vi "Save ALL Contacts.vi"(6 "Command":T8=enum."Set Position", 8 "error in (no error)":errorcluster, 11 "Contact in":T1[](array[typedef])) -> (0 "error out":errorcluster, 3 "Contact out":T1[](array[typedef]))   [LabVIEW 2014, in "Contact Data.lvlib"]
doc: "Updates an existing contact or inserts a new contact into the address book data store. Use the ID of an existing contact to update, or an ID of 0 to insert. When inserting, the output cluster will contain the ID of the new contact."
uses:
  Contact Data.lvlib
  Command.ctl
  Contact.ctl
  Position.ctl
  Controls.ctl
  DestinationCluster.ctl
  DesinationControls.ctl
  PathData.ctl
  Components/PathFinder/Controls/PathControl.ctl
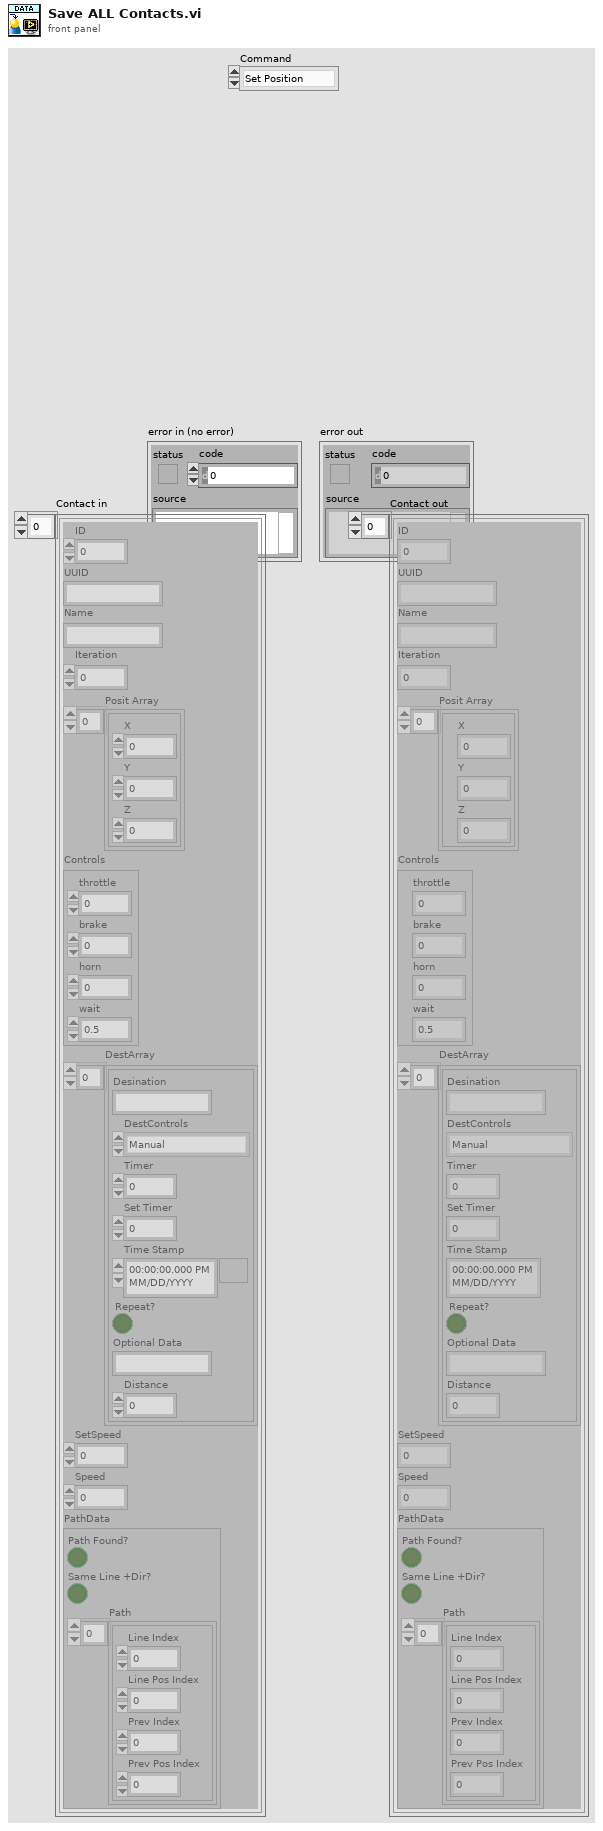
[diagram p1: front panel]
types:
  T1 = typedef "Contact Data.lvlib/Contact.ctl" = cluster{"ID":u32, "UUID":string, "Name":string, "Iteration":i32, "Posit Array":T2[], "Controls":T3, "DestArray":T4[], "SetSpeed":dbl, "Speed":dbl, "PathData":T6}
  T2 = typedef "Contact Data.lvlib/Position.ctl" = cluster{"X":dbl, "Y":dbl, "Z":dbl}
  T3 = typedef "Contact Data.lvlib/Controls.ctl" = cluster{"throttle":dbl, "brake":dbl, "horn":dbl, "wait":dbl}
  T4 = typedef "Contact Data.lvlib/DestinationCluster.ctl" = cluster{"Desination":string, "DestControls":T5, "Timer":u32, "Set Timer":u32, "Time Stamp":timestamp, "Repeat?":bool, "Optional Data":string, "Distance":dbl}
  T5 = typedef "Contact Data.lvlib/DesinationControls.ctl" = enum16{"Tracker", "Manual", "Stop", "Station DateTime", "Station Timer", "Maintain"}
  T6 = typedef "Contact Data.lvlib/PathData.ctl" = cluster{"Path Found?":bool, "Same Line +Dir?":bool, "Path":T7[]}
  T7 = typedef "PathControl.ctl" = cluster{"Line Index":i32, "Line Pos Index ":i32, "Prev Index ":i32, "Prev Pos Index":i32}
  T8 = typedef "Contact Data.lvlib/Command.ctl" = enum16{"Set All Contacts", "Load", "Save", "Get All Data", "Get Single Data (ID)", "Get Single Data", "Set Position", "Set Destinations", "Set Controls", "Remove Single Data", "Remove UUID Contact", "Set Single ALL", "Is Data Modified", "Import Data"}
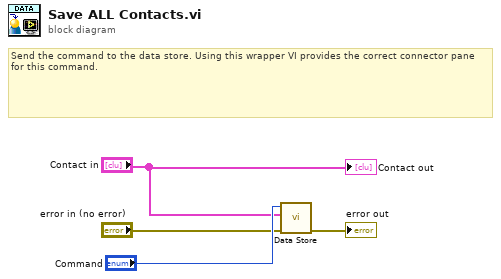
[diagram p0: block diagram]
diagram:
  # "Send the command to the data store. Using this wrapper VI provides the correct connector pane for this command."
  n1 = call "Data Store.vi"("error in (no error)"="error in (no error)", "Contact in"="Contact in", "Command"="Command") -> ("error out"=→"error out":errorcluster)  [unwired: 6 in, 2 out]
  "Contact out" <- "Contact in"
